vi "Regex_LoopArray.vi"(8 "error in":errorcluster, 10 "regular expression":string="^([\\d]{4})([-\\/.])(0[1-9]|1[012])\\2(0[1-9]|[12][0-9]|3[01])", 11 "String-Array (In)":string[](array[string])) -> (0 "Error Out":errorcluster)   [LabVIEW 2017] (continued)
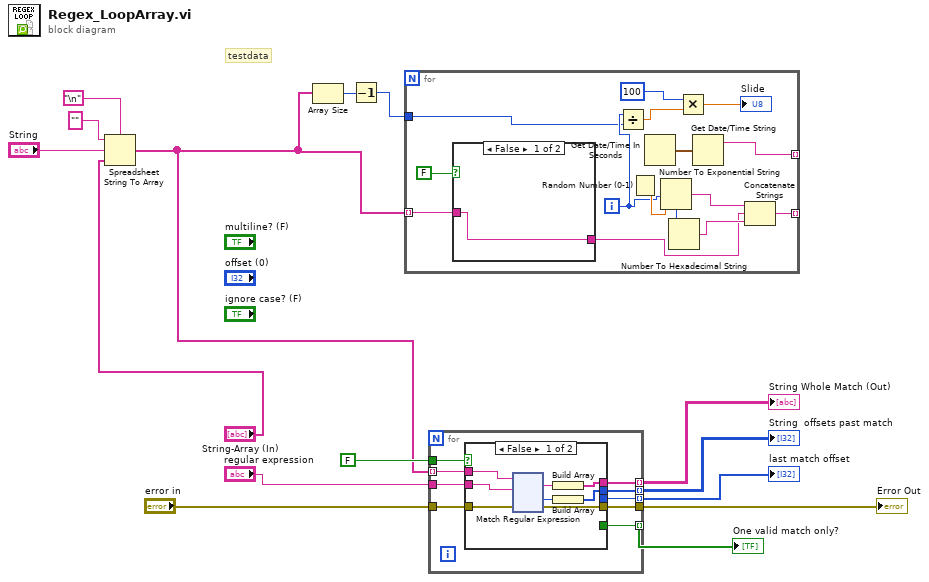
[diagram p0: block diagram]
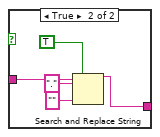
[diagram p2: hidden frame]
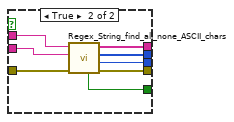
[diagram p3: hidden frame]
diagram:
  # "testdata"
  n1 = Spreadsheet String To Array(delimiter (Tab)="\n", format string="", spreadsheet string="String", array type (2D Dbl)="String-Array (In)") -> (array=w1:string[])
  n2 = Array Size(array=w1) -> (size(s)=w4:i32)
  n3 = Decrement(x=w4) -> (x-1=w3:i32)
  n4 = for {
    tunnel: [w28] -> _ mode=indexing
    tunnel: w1 -> [w23] mode=indexing
    tunnel: [w24] -> _ mode=indexing
    tunnel: w3 -> [w17]
    i -> [w20]
    n5 = case shown="False" FALSE ("replace all? (F)") {
      tunnel: w23 -> [w30 w35]
      tunnel: [w30 w31] -> w22
      frame False {
      }
      frame True {
        n6 = Search and Replace String(replace all?=TRUE ("replace all? (F)"), input string=w35, search string=".", replace string="" ("replace string (\"\")")) -> (result string=w31:string)  [unwired: 4 in, 3 out]
      }
    }
    n7 = Divide(x=w20, y=w17) -> (x/y=w19:dbl)
    n8 = Random Number (0-1)() -> (number: 0 to 1=w27:dbl)
    n9 = Get Date/Time In Seconds() -> (seconds since 1Jan1904=w29:timestamp)
    n10 = Number To Exponential String(number=w27) -> (E-format string=w26:string)  [unwired: 3 in]
    n11 = Number To Hexadecimal String(2:w20) -> (0:w25:string)  [unwired: 1 in]
    n12 = Multiply(x=100, y=w19) -> (x*y=→"Slide":dbl)
    n13 = Get Date/Time String(seconds (now)=w29) -> (date string=w28:string)  [unwired: 2 in, 1 out]
    n14 = Concatenate Strings(w26, w22, w25) -> (w24:string)
  }
  n15 = for {
    tunnel: [w44] -> w15 mode=indexing
    tunnel: [w39] -> w14 mode=indexing
    tunnel: [w43] -> w13 mode=indexing
    tunnel: "error in" -> [w42]
    tunnel: [w41] -> w11
    tunnel: [w40] -> w10 mode=indexing
    tunnel: w1 -> [w38] mode=indexing
    tunnel: FALSE ("replace all? (F)") -> [w37]
    tunnel: "regular expression" -> [w36]
    n16 = case shown="False" w37 {
      tunnel: [_ w174] -> w44
      tunnel: [_ w173] -> w43
      tunnel: w42 -> [w47 w172]
      tunnel: [w46 w171] -> w41
      tunnel: [w51 w170] -> w40
      tunnel: [w48 w169] -> w39
      tunnel: w38 -> [w52 w168]
      tunnel: w36 -> [w45 w167]
      frame False {
        n17 = xnode "Match Regular Expression"("input string"=w52, "regular expression"=w45, "error in"=w47) -> ("whole match"=w50:string, "offset past match"=w49:i32, "error out"=w46:errorcluster)  [unwired: 3 in, 2 out]
        n18 = Build Array(w50) -> (w51:string[])
        n19 = Build Array(w49) -> (w48:i32[])
      }
      frame True {
        n20 = call "Regex_String_find_all_none_ASCII_chars.vi"("Error In"=w172, "Regex"=w167, "String (In)"=w168) -> ("Error Out"=w171:errorcluster, "last match offset"=w174:i32, "offsets past match"=w169:i32[], "Whole Match"=w170:string[], "One valid match only?"=w173:bool)  [unwired: 4 in]
      }
    }
  }
  "last match offset" <- w15
  "String  offsets past match" <- w14
  "String Whole Match (Out)" <- w10
  "One valid match only?" <- w13
  "Error Out" <- w11
